vi "FPGAmain_5782_utanFIFO.vi"() -> ()   [LabVIEW 2013]
uses:
  FPGA/DataMode.ctl
  FPGA/Input_5782/5782_states.ctl
  <vilib>/Platform/TimedLoop/XDataNode/timing_clust.ctl
  <vilib>/Platform/TimedLoop/XDataNode/nitl_modes.ctl
  <vilib>/Platform/TimedLoop/XDataNode/wakeup.ctl
  <vilib>/rvi/Emulation/niFpgaSctlEmulationGetInTimedLoop.vi
  <vilib>/rvi/Emulation/niFpgaEmulationReportErrorSimple.vi
  <vilib>/rvi/Emulation/niFpgaGetClockAttributes.vi
  <vilib>/rvi/eio/common/nirviEmuTemplateMethod_errors.vi
  <vilib>/rvi/Emulation/niFpgaCriticalErrorInLSC.vi
  <vilib>/rvi/DataTransferAndStorage/Register/Emulation/niFpgaRegisterEmulationFpgaImpl.vi
  <instcachedir>/0/niFpgaRegisterEmulationFpgaImpl_DCF4BC0110594B98B44A971D60CEEC4D.lvgen/niFpgaRegisterEmulationFpgaImpl_DCF4BC0110594B98B44A971D60CEEC4D_017.vi
  <vilib>/rvi/DataTransferAndStorage/Container/Common/niFpgaContainerGetUniqueNameForEmu.vi
  <instcachedir>/0/niFpgaRegisterEmulationFpgaImpl_DCF4BC0110594B98B44A971D60CEEC4D.lvgen/niFpgaRegisterEmulationFpgaImpl_DCF4BC0110594B98B44A971D60CEEC4D_003.vi
  <instcachedir>/0/niFpgaRegisterEmulationFpgaImpl_DCF4BC0110594B98B44A971D60CEEC4D.lvgen/niFpgaRegisterEmulationFpgaImpl_DCF4BC0110594B98B44A971D60CEEC4D_016.vi
  <instcachedir>/0/niFpgaRegisterEmulationFpgaImpl_DCF4BC0110594B98B44A971D60CEEC4D.lvgen/niFpgaRegisterEmulationFpgaImpl_DCF4BC0110594B98B44A971D60CEEC4D_010.vi
  <instcachedir>/0/niFpgaRegisterEmulationFpgaImpl_DCF4BC0110594B98B44A971D60CEEC4D.lvgen/niFpgaRegisterEmulationFpgaImpl_DCF4BC0110594B98B44A971D60CEEC4D_011.vi
  <instcachedir>/0/niFpgaRegisterEmulationFpgaImpl_DCF4BC0110594B98B44A971D60CEEC4D.lvgen/niFpgaRegisterEmulationFpgaImpl_DCF4BC0110594B98B44A971D60CEEC4D_012.vi
  <instcachedir>/0/niFpgaRegisterEmulationFpgaImpl_DCF4BC0110594B98B44A971D60CEEC4D.lvgen/niFpgaRegisterEmulationFpgaImpl_DCF4BC0110594B98B44A971D60CEEC4D_009.vi
  <vilib>/rvi/interface/RandomDataEmulation/nirviRandomDataMultiElementFPGAFIFO.vi
  <instcachedir>/0/nirviRandomDataMultiElementFPGAFIFO_F2B80EDE0D7944A08478D8D26097D4DB.lvgen/nirviRandomDataMultiElementFPGAFIFO_F2B80EDE0D7944A08478D8D26097D4DB_005.vi
  <vilib>/rvi/interface/RandomDataEmulation/niFpgaRandomDataHandleErrors.vi
  <instcachedir>/0/niFpgaRegisterEmulationFpgaImpl_DCF4BC0110594B98B44A971D60CEEC4D.lvgen/niFpgaRegisterEmulationFpgaImpl_DCF4BC0110594B98B44A971D60CEEC4D_013.vi
  <vilib>/rvi/interface/RandomDataEmulation/nirviRandomDataFPGAFIFO.vi
  <instcachedir>/0/niFpgaRegisterEmulationFpgaImpl_DCF4BC0110594B98B44A971D60CEEC4D.lvgen/niFpgaRegisterEmulationFpgaImpl_DCF4BC0110594B98B44A971D60CEEC4D_018.vi
  <instcachedir>/0/niFpgaRegisterEmulationFpgaImpl_DCF4BC0110594B98B44A971D60CEEC4D.lvgen/niFpgaRegisterEmulationFpgaImpl_DCF4BC0110594B98B44A971D60CEEC4D_019.vi
  <vilib>/Platform/TimedLoop/XDataNode/XDataNode.xnode
  <vilib>/eio/EIONode/EIONode.xnode
  <vilib>/rvi/DataTransferAndStorage/Container/XNode/niFpgaContainer.xnode
  <vilib>/rvi/DataTransferAndStorage/Register/Emulation/niFpgaRegisterEmulation.vi
  <vilib>/rvi/interface/RandomDataEmulation/nirviRandomDataFpgaMultiElementTemplate.vi
  <vilib>/rvi/interface/RandomDataEmulation/nirviRandomDataFpgaReadWriteTemplate.vi
  <vilib>/Platform/TimedLoop/XDataNode/XDNodeRunTimeDep.lvlib
  <vilib>/rvi/FIFO/Fifo_Resource/nirvififoEmulationRead.vi
  <vilib>/rvi/FIFO/Fifo_Resource/nirvififoEmulationWrite.vi
panel:
  in  "Data array":fxp<+/-,16,14>[](array[numeric])=[0.0, 0.0, 0.0, 0.0]
  in  "AM phase":fxp<+,64,64>
  in  "delay phase":fxp<+,64,64>
  in  "User Command Commit":bool
  in  "User Command":u8
  out "User Command Idle":bool
  out "User Command Status":u8
  in  "User Data 0":u8
  in  "User Data 1":u8
  out "PLL Locked":bool
  out "User Error":bool
  out "Configured?":bool
  in  "Continuous":bool
  in  "5782 record length":u16=4000 caption="Samples Per Trigger" min=1 step=1
  in  "Trigger Acquisition":bool
  out "IO Module\\Trigger Input":bool
  in  "Downsample":fxp<+,8,8>=1.0
  in  "new coeffs":bool
  in  "FIR coeffs":fxp<+/-,18,18>[](array[numeric])
  in  "CIC Gain":fxp<+/-,32,1>=0.00390625 format="%#_32g"
  in  "Acquisition running":bool
  in  "Phase output":fxp<+,64,64>[](array[numeric])=[0.0, 0.0, 0.0, 0.0, 0.0, 0.0, 0.0, 0.0]
  in  "Simulated phase 5782":fxp<+,64,64>[](array[numeric])=[0.0, 0.0]
  in  "Mode":T1
  in  "Phase 5782":fxp<+,64,64>[](array[numeric])=[0.0, 0.0]
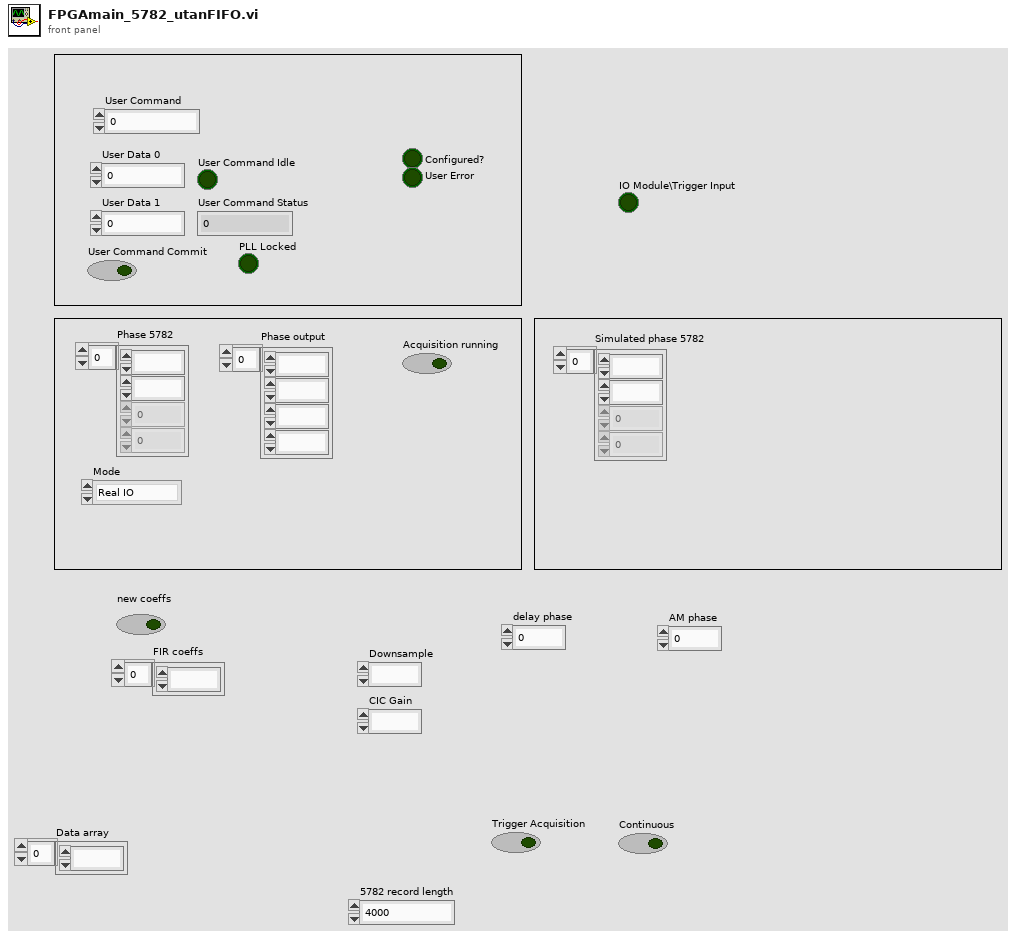
[diagram p1: front panel]
types:
  T1 = typedef "DataMode.ctl" = enum16{"Real IO", "Simulated"}
  T2 = typedef "5782_states.ctl" = enum8{"Wait for trigger", "Acquisition", "Send record length", "Quiet period"}
  T3 = typedef "XDNodeRunTimeDep.lvlib/timing_clust.ctl" = cluster{"Expected End [f-1]":u64, "Actual End [f-1]":u64, "Finished Late? [f-1]":bool, "Expected End [i-1]":u64, "Actual End [i-1]":u64, "Finished Late? [i-1]":bool, "Expected Start [i]":u64, "Actual Start [i]":u64, "Expected Start [f]":u64, "Actual Start [f]":u64, "Source Name":string, "Structure Name":string, "Period":i64, "Deadline":i64, "Offset":i64, "Start":i64, "Priority":i32, "Timeout":i32, "Mode":T4, "Wakeup Reason":T5, "Error":errorcluster, "Source Type":string, "Secondary Source Type":string, "Global End Time":u64, "Global Start Time":u64, "Frame Duration":u64, "Iteration Duration":u64, "Assigned CPU":i32, "I/O Scan Engine Mode":u32}
  T4 = typedef "XDNodeRunTimeDep.lvlib/nitl_modes.ctl" = enum32{"No Change", "Process missed periods, maintain original phase", "Discard missed periods, maintain original phase", "Process missed periods, ignore original phase", "Discard missed periods, ignore original phase"}
  T5 = typedef "XDNodeRunTimeDep.lvlib/wakeup.ctl" = enum32{"Normal", "Aborted", "Asynchronous wakeup", "Timing source error", "Timed loop error", "Timeout"}
  T6 = typedef "I16 array size 2.ctl" = i16[]
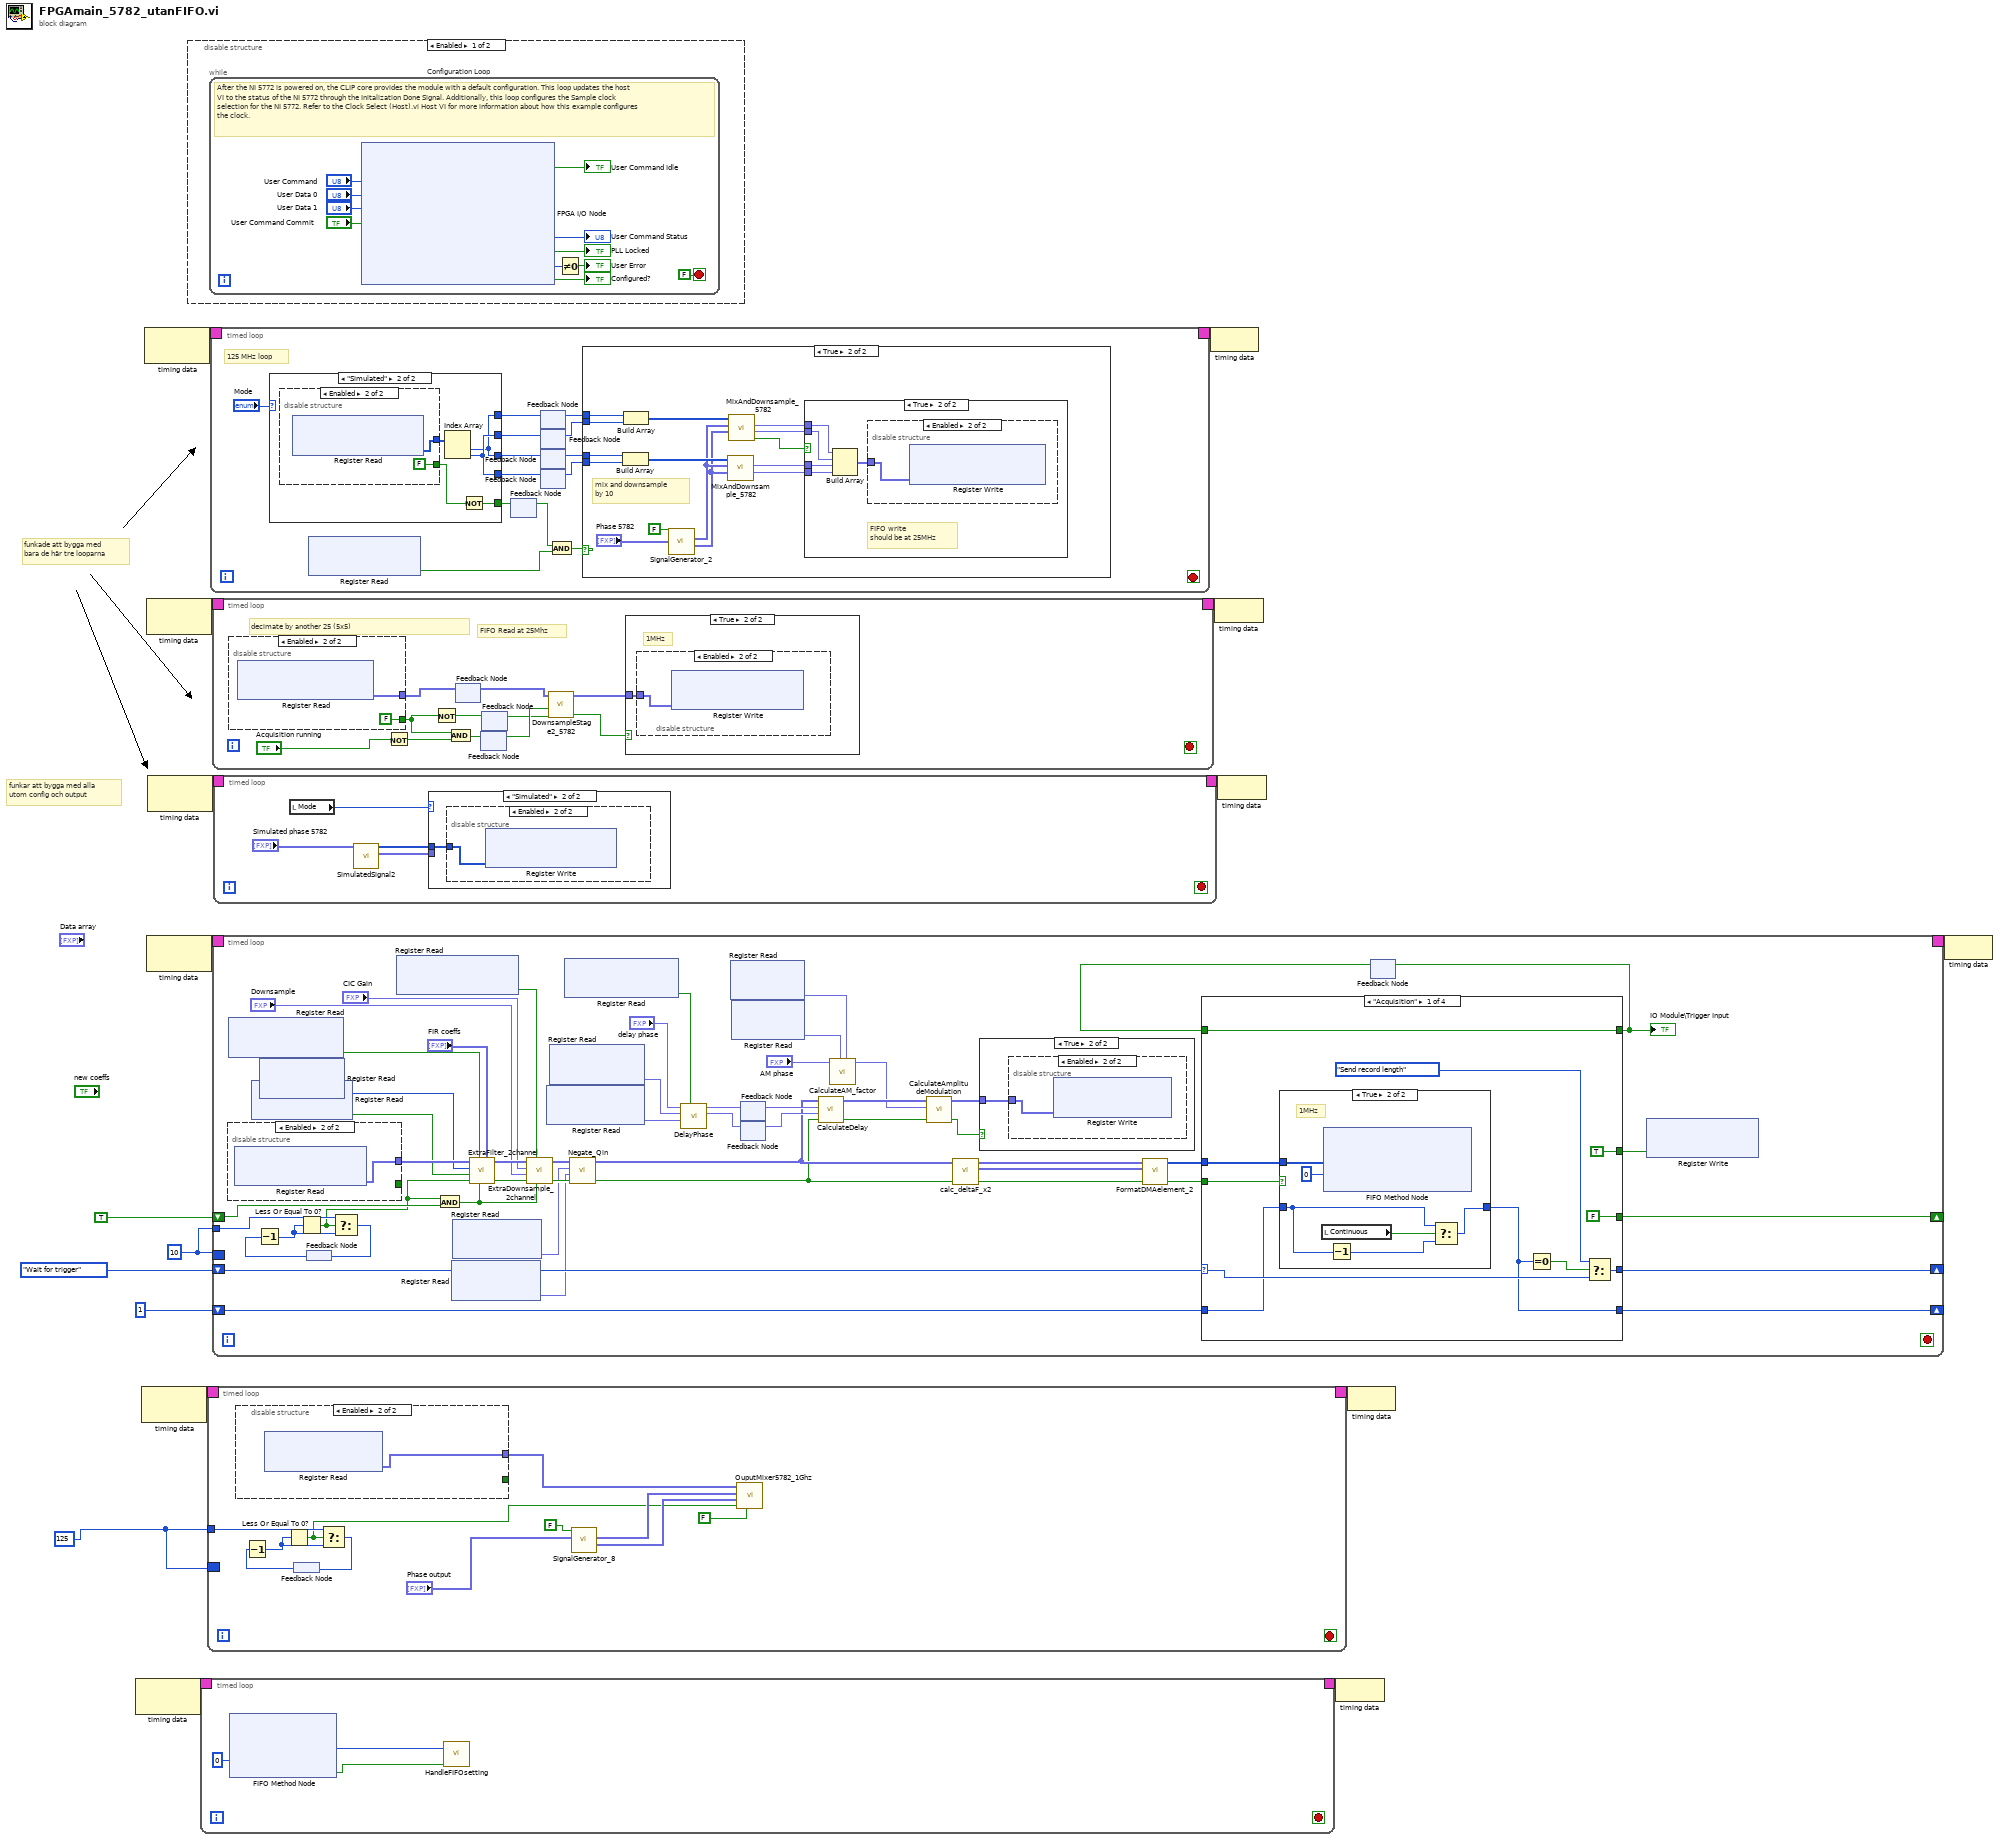
[diagram p0: block diagram]
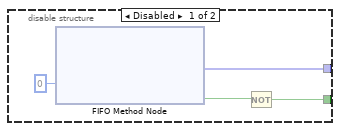
[diagram p2: hidden frame]
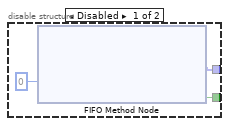
[diagram p3: hidden frame]
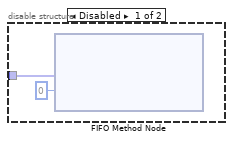
[diagram p5: hidden frame]
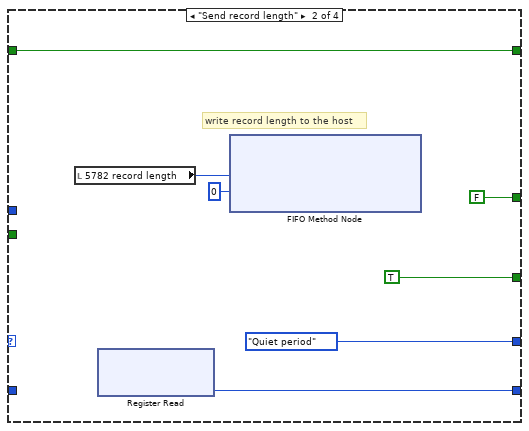
[diagram p7: hidden frame]
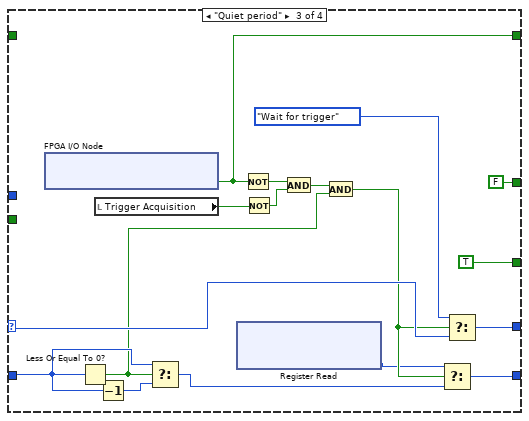
[diagram p8: hidden frame]
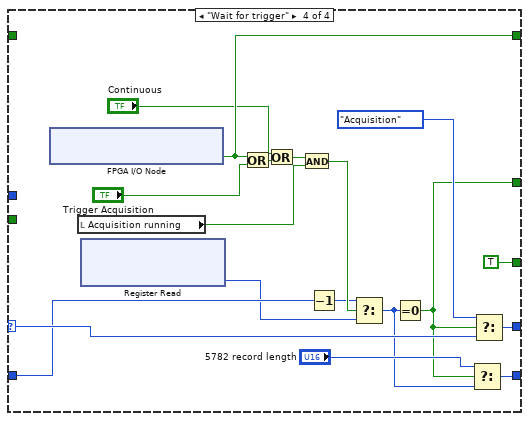
[diagram p9: hidden frame]
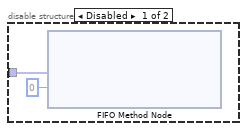
[diagram p13: hidden frame]
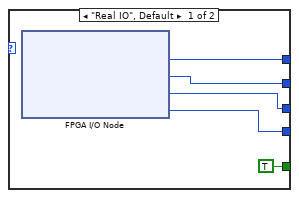
[diagram p14: hidden frame]
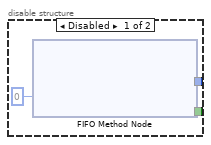
[diagram p15: hidden frame]
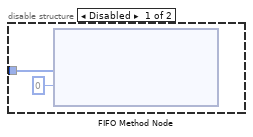
[diagram p17: hidden frame]
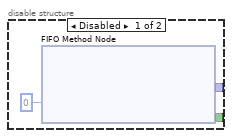
[diagram p18: hidden frame]
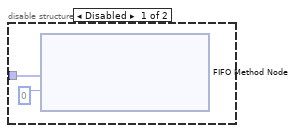
[diagram p20: hidden frame]
diagram:
  w1 = u8 125 ("trigger samples")
  w2 = u8 10 ("trigger samples")
  # "funkar att bygga med alla\nutom config och output"
  # "funkade att bygga med\nbara de här tre looparna"
  n1 = node-c288() -> (w6:T3)  [unwired: 1 in]
  n2 = node-c288() -> (w4:T3)  [unwired: 1 in]
  n3 = node-c288() -> (w13:T3)  [unwired: 1 in]
  n4 = node-c288() -> (w17:T3)  [unwired: 1 in]
  n5 = node-c288() -> (w11:T3)  [unwired: 1 in]
  n6 = node-c288() -> (w15:T3)  [unwired: 1 in]
  n7 = disable-structure shown="Enabled" {
    frame Enabled {
      n8 = while "Configuration Loop" {
        stop <- FALSE stop-if-true
        # "After the NI 5772 is powered on, the CLIP core provides the module with a default configuration. This loop updates the host VI to the status of the NI 5772 through the Initalization Done Signal. Additionally, this loop configures the Sample clock selection for the NI 5772. Refer to the Clock Select (Host).vi Host VI for more information about how this example configures the clock."
        n9 = xnode "FPGA I/O Node"("IO Module\\User Command"="User Command", "IO Module\\User Data 0"="User Data 0", "IO Module\\User Data 1"="User Data 1", "IO Module\\User Command Commit"="User Command Commit") -> ("IO Module\\User Command Idle"=→"User Command Idle":bool, "IO Module\\User Command Status"=→"User Command Status":u8, "IO Module\\PLL Locked"=→"PLL Locked":bool, "IO Module\\User Error"=w23:u8, "IO Module\\Initialization Done"=→"Configured?":bool)  [unwired: 9 in, 9 out]
        n10 = Not Equal To 0?(x=w23) -> (x != 0?=→"User Error":bool)
      }
    }
    frame Disabled {
    }
  }
  n11 = timed-loop {
    timing: w6 -> [_]
    timing-out: [_] -> w5
    stop <- _ stop-if-true
    n12 = xnode ("FIFO Method Node")("Timeout"=0) -> ("Element"=w30:u64, "Timed Out?"=w29:bool)  [unwired: 1 in, 1 out]
    n13 = call "HandleFIFOsetting.vi"("timed out"=w29, "Value"=w30) -> ()  [unwired: 10 in]
  }
  n14 = timed-loop {
    timing: w4 -> [_]
    timing-out: [_] -> w3
    tunnel: w1 -> [w38]
    border: w1 -> [_]
    stop <- _ stop-if-true
    n15 = disable-structure shown="Enabled" {
      disable-tunnel: [w47 w49] -> w42
      disable-tunnel: [w45 _] -> _
      frame Disabled {
        n16 = xnode ("FIFO Method Node")("Timeout"=0) -> ("Element"=w47:fxp<+/-,16,14>[], "Timed Out?"=w46:bool)  [unwired: 1 in, 1 out]
        n17 = Not(x=w46) -> (.not. x?=w45:bool)
      }
      frame Enabled {
        n18 = xnode ("Register Read")() -> ("Data"=w49:fxp<+/-,16,14>[])  [unwired: 1 in, 1 out]
      }
    }
    n19 = feedback #1() -> (w36:u8)
    n20 = Decrement(x=w36) -> (x-1=w34:u8)
    n21 = Less Or Equal To 0?(x=w34) -> (x <= 0?=w35:bool)
    n22 = Select(t=w38, s=w35, f=w34) -> (s? t:f=w37:u8)
    n23 = feedback-in #1(w37) -> ()
    n24 = call "SignalGenerator_8.vi"("Phase"="Phase output", "reset"=FALSE) -> ("Sine out"=w39:fxp<+/-,16,0>[], "Cosine out"=w40:fxp<+/-,16,0>[])  [unwired: 8 in]
    n25 = call "OuputMixer5782_1Ghz.vi"("reset"=FALSE, "valid in"=w35, "Sine in"=w39, "Cosine in"=w40, "Data in"=w42) -> ()  [unwired: 5 in, 2 out]
  }
  n26 = timed-loop {
    timing: w13 -> [_]
    timing-out: [_] -> w12
    stop <- _ stop-if-true
    # "125 MHz loop"
    n27 = case shown="\"Simulated\"" "Mode" {
      tunnel: [w92 w95] -> w62
      tunnel: [w91 w96] -> w60
      tunnel: [w90 w95] -> w58
      tunnel: [w89 w96] -> w55
      tunnel: [TRUE w93] -> w54
      frame "Real IO", Default {
        n28 = xnode "FPGA I/O Node"() -> ("IO Module\\AI 0 N-1"=w92:i16, "IO Module\\AI 0 N"=w91:i16, "IO Module\\AI 1 N-1"=w90:i16, "IO Module\\AI 1 N"=w89:i16)  [unwired: 4 in, 4 out]
      }
      frame "Simulated" {
        n29 = disable-structure shown="Enabled" {
          disable-tunnel: [w99 w102] -> w97
          disable-tunnel: [w98 FALSE ("Timed Out?")] -> w94
          frame Disabled {
            n30 = xnode ("FIFO Method Node")("Timeout"=0) -> ("Element"=w99:i16[], "Timed Out?"=w98:bool)  [unwired: 1 in, 1 out]
          }
          frame Enabled {
            n31 = xnode "Register Read"() -> ("Data"=w102:i16[])  [unwired: 1 in, 1 out]
          }
        }
        n32 = Index Array(array=w97) -> (element #1=w95:i16, element #2=w96:i16)  [unwired: 2 in]
        n33 = Not(x=w94) -> (.not. x?=w93:bool)
      }
    }
    n34 = xnode ("Register Read")() -> ("Data"=w52:bool)  [unwired: 1 in, 1 out]
    n35 = feedback #2() -> (w53:bool)  [unwired: 1 in]
    n36 = feedback-in #2(w54) -> ()
    n37 = feedback #3() -> (w61:i16)  [unwired: 1 in]
    n38 = feedback-in #3(w62) -> ()
    n39 = feedback #4() -> (w59:i16)  [unwired: 1 in]
    n40 = feedback-in #4(w60) -> ()
    n41 = feedback #5() -> (w57:i16)  [unwired: 1 in]
    n42 = feedback-in #5(w58) -> ()
    n43 = feedback #6() -> (w56:i16)  [unwired: 1 in]
    n44 = feedback-in #6(w55) -> ()
    n45 = And(x=w53, y=w52) -> (x .and. y?=w63:bool)
    n46 = case shown="True" w63 {
      tunnel: w61 -> [_ w70]
      tunnel: w59 -> [_ w69]
      tunnel: w57 -> [_ w68]
      tunnel: w56 -> [_ w67]
      frame False {
      }
      frame True {
        # "mix and downsample\nby 10"
        n47 = Build Array(w68, w67) -> (w79:i16[])
        n48 = Build Array(w70, w69) -> (w66:i16[])
        n49 = call "SignalGenerator_2.vi"("Phase"="Phase 5782", "reset"=FALSE) -> ("Sine out"=w71:fxp<+/-,16,0>[], "Cosine out"=w72:fxp<+/-,16,0>[])  [unwired: 8 in]
        n50 = call "MixAndDownsample_5782.vi"("Sine in"=w71, "Cosine in"=w72, "Signal Input"=w79) -> ("Q out"=w74:fxp<+/-,16,14>, "I out"=w75:fxp<+/-,16,14>)  [unwired: 6 in, 1 out]
        n51 = call "MixAndDownsample_5782.vi"("Sine in"=w71, "Cosine in"=w72, "Signal Input"=w66) -> ("data valid"=w76:bool, "Q out"=w77:fxp<+/-,16,14>, "I out"=w78:fxp<+/-,16,14>)  [unwired: 6 in]
        n52 = case shown="True" w76 {
          tunnel: w77 -> [_ w84]
          tunnel: w78 -> [_ w82]
          tunnel: w75 -> [_ w81]
          tunnel: w74 -> [_ w80]
          frame False {
          }
          frame True {
            # "FIFO write\nshould be at 25MHz"
            n53 = Build Array(w82, w84, w81, w80) -> (w83:fxp<+/-,16,14>[])
            n54 = disable-structure shown="Enabled" {
              disable-tunnel: w83 -> [w86 w87]
              frame Disabled {
                n55 = xnode ("FIFO Method Node")("Element"=w86, "Timeout"=0) -> ()  [unwired: 1 in, 2 out]
              }
              frame Enabled {
                n56 = xnode ("Register Write")("Data"=w87) -> ()  [unwired: 1 in, 1 out]
              }
            }
          }
        }
      }
    }
  }
  n57 = timed-loop {
    timing: w17 -> [_]
    timing-out: [_] -> w16
    stop <- _ stop-if-true
    # "FIFO Read at 25Mhz"
    # "decimate by another 25 (5x5)"
    n58 = disable-structure shown="Enabled" {
      disable-tunnel: [w117 FALSE ("Timed Out?")] -> w112
      disable-tunnel: [w116 w120] -> w110
      frame Disabled {
        n59 = xnode ("FIFO Method Node")("Timeout"=0) -> ("Element"=w116:fxp<+/-,16,14>[], "Timed Out?"=w117:bool)  [unwired: 1 in, 1 out]
      }
      frame Enabled {
        n60 = xnode ("Register Read")() -> ("Data"=w120:fxp<+/-,16,14>[])  [unwired: 1 in, 1 out]
      }
    }
    n61 = Not(x="Acquisition running") -> (.not. x?=w113:bool)
    n62 = Not(x=w112) -> (.not. x?=w106:bool)
    n63 = And(x=w112, y=w113) -> (x .and. y?=w108:bool)
    n64 = feedback #7() -> (w109:fxp<+/-,16,14>[])  [unwired: 1 in]
    n65 = feedback-in #7(w110) -> ()
    n66 = feedback #8() -> (w107:bool)  [unwired: 1 in]
    n67 = feedback-in #8(w108) -> ()
    n68 = feedback #9() -> (w105:bool)  [unwired: 1 in]
    n69 = feedback-in #9(w106) -> ()
    n70 = call "DownsampleStage2_5782.vi"("valid in"=w105, "reset"=w107, "Data in"=w109) -> ("valid out"=w114:bool, "data out"=w115:fxp<+/-,16,14>[])  [unwired: 7 in]
    n71 = case shown="True" w114 {
      tunnel: w115 -> [_ w121]
      frame False {
      }
      frame True {
        # "1MHz"
        n72 = disable-structure shown="Enabled" {
          disable-tunnel: w121 -> [w122 w124]
          frame Disabled {
            n73 = xnode ("FIFO Method Node")("Element"=w122, "Timeout"=0) -> ()  [unwired: 1 in, 2 out]
          }
          frame Enabled {
            n74 = xnode ("Register Write")("Data"=w124) -> ()  [unwired: 1 in, 1 out]
          }
        }
      }
    }
  }
  n75 = timed-loop {
    timing: w11 -> [_]
    timing-out: [_] -> w10
    shift-right: [w176] -> _
    shift-left: 5782_states."Wait for trigger" ("5782 states") -> [w178]
    shift-right: [w175] -> _
    shift-left: u16 1 ("trigger samples") -> [w177]
    shift-right: [w164] -> _
    shift-left: TRUE -> [w167]
    border: w2 -> [_]
    tunnel: w2 -> [w130]
    stop <- _ stop-if-true
    n76 = disable-structure shown="Enabled" {
      disable-tunnel: [w180 w182] -> w168
      disable-tunnel: [w179 _] -> _
      frame Disabled {
        n77 = xnode ("FIFO Method Node")("Timeout"=0) -> ("Element"=w180:fxp<+/-,16,14>[], "Timed Out?"=w179:bool)  [unwired: 1 in, 1 out]
      }
      frame Enabled {
        n78 = xnode ("Register Read")() -> ("Data"=w182:fxp<+/-,16,14>[])  [unwired: 1 in, 1 out]
      }
    }
    n79 = xnode ("Register Read")() -> ("Data"=w142:bool)  [unwired: 1 in, 1 out]
    n80 = xnode ("Register Read")() -> ("Data"=w132:bool)  [unwired: 1 in, 1 out]
    n81 = xnode ("Register Read")() -> ("Data"=w133:i32)  [unwired: 1 in, 1 out]
    n82 = feedback #10() -> (w131:u8)
    n83 = Decrement(x=w131) -> (x-1=w129:u8)
    n84 = Less Or Equal To 0?(x=w129) -> (x <= 0?=w127:bool)
    n85 = Select(t=w130, s=w127, f=w129) -> (s? t:f=w128:u8)
    n86 = feedback-in #10(w128) -> ()
    n87 = xnode ("Register Read")() -> ("Data"=w134:bool)  [unwired: 1 in, 1 out]
    n88 = And(x=w127, y=w167) -> (x .and. y?=w174:bool)
    n89 = xnode ("Register Read")() -> ("Data"=w140:fxp<+/-,16,14>)  [unwired: 1 in, 1 out]
    n90 = xnode ("Register Read")() -> ("Data"=w141:fxp<+/-,16,14>)  [unwired: 1 in, 1 out]
    n91 = call "ExtraFilter_2channel.vi"(5:"new coeffs"="FIR coeffs", "reset"=w174, 7:"new coeffs"=w142, "valid in"=w127, "enable filter"=w132, "new shift"=w133, "Data in"=w168) -> ("valid out"=w173:bool, "Data out"=w172:fxp<+/-,16,14>[])  [unwired: 3 in]
    n92 = call "ExtraDownsample_2channel.vi"("reset"=w174, "Set downsample"=w134, "valid in"=w173, "Downsample"="Downsample", "CIC Gain"="CIC Gain", "Data in"=w172) -> ("valid out"=w159:bool, "Data out"=w160:fxp<+/-,16,14>[])  [unwired: 4 in]
    n93 = xnode ("Register Read")() -> ("Data"=w135:fxp<+/-,16,0>)  [unwired: 1 in, 1 out]
    n94 = xnode ("Register Read")() -> ("Data"=w136:fxp<+/-,16,0>)  [unwired: 1 in, 1 out]
    n95 = xnode ("Register Read")() -> ("Data"=w137:bool)  [unwired: 1 in, 1 out]
    n96 = call "Negate_Qin.vi"("valid in"=w159, "DC offset chan 1"=w140, "DC offset chan 0"=w141, "Data in"=w160) -> ("valid out"=w145:bool, "Data out"=w151:fxp<+/-,16,14>[])  [unwired: 6 in]
    n97 = call "DelayPhase.vi"("Use fixed delay"=w137, "fixed cos_fi"=w135, "fixed sin fi"=w136, "delay phase"="delay phase") -> ("cos_fi"=w148:fxp<+/-,16,0>, "sin fi"=w149:fxp<+/-,16,0>)  [unwired: 6 in]
    n98 = xnode ("Register Read")() -> ("Data"=w139:fxp<+/-,16,2>)  [unwired: 1 in, 1 out]
    n99 = xnode ("Register Read")() -> ("Data"=w138:fxp<+/-,16,2>)  [unwired: 1 in, 1 out]
    n100 = feedback-in #11(w149) -> ()
    n101 = feedback #11() -> (w158:fxp<+/-,16,0>)  [unwired: 1 in]
    n102 = feedback #12() -> (w157:fxp<+/-,16,0>)  [unwired: 1 in]
    n103 = feedback-in #12(w148) -> ()
    n104 = call "CalculateDelay.vi"("input valid"=w145, "cos_fi"=w157, "sin fi"=w158, "Data in"=w151) -> ("output valid"=w155:bool, "Data out"=w156:fxp<+/-,16,14>[])  [unwired: 6 in]
    n105 = call "CalculateAM_factor.vi"("b_am"=w139, "a_am"=w138, "AM phase"="AM phase") -> ("AM_factor"=w152:fxp<+/-,16,2>)  [unwired: 7 in, 1 out]
    n106 = call "CalculateAmplitudeModulation.vi"("input valid"=w155, "AM_factor"=w152, "Data in"=w156) -> ("output valid"=w153:bool, "Data out"=w154:fxp<+/-,16,14>[])  [unwired: 7 in]
    n107 = call "calc_deltaF_x2.vi"("valid in"=w145, "Data in"=w151) -> ("valid out"=w144:bool, "deltaF"=w143:fxp<+/-,32,30>[], "Data out"=w146:fxp<+/-,16,14>[])  [unwired: 7 in]
    n108 = case shown="True" w153 {
      tunnel: w154 -> [_ w183]
      frame False {
      }
      frame True {
        n109 = disable-structure shown="Enabled" {
          disable-tunnel: w183 -> [w184 w186]
          frame Disabled {
            n110 = xnode ("FIFO Method Node")("Element"=w184, "Timeout"=0) -> ()  [unwired: 1 in, 2 out]
          }
          frame Enabled {
            n111 = xnode ("Register Write")("Data"=w186) -> ()  [unwired: 1 in, 1 out]
          }
        }
      }
    }
    n112 = call "FormatDMAelement_2.vi"("valid in"=w144, "deltaF"=w143, "Data in"=w146) -> ("valid out"=w165:bool, "Element"=w166:u64[])  [unwired: 7 in]
    n113 = feedback #13() -> (w162:bool)  [unwired: 1 in]
    n114 = case shown="\"Acquisition\"" w178 {
      selector: w178 -> [w197 _ w227 w246]
      tunnel: w177 -> [w193 _ w215 w233]
      tunnel: [w196 5782_states."Quiet period" ("5782 states") w226 w245] -> w176
      tunnel: [w190 w205 w228 w244] -> w175
      tunnel: w166 -> [w191 _ _ _]
      tunnel: w165 -> [w192 _ _ _]
      tunnel: [FALSE TRUE TRUE TRUE] -> w164
      tunnel: [TRUE FALSE ("5782 triggered") FALSE ("5782 triggered") w237] -> w163
      tunnel: [w189 w206 w217 w236] -> w161
      tunnel: w162 -> [w189 w206 _ _]
      frame "Acquisition" {
        n115 = case shown="True" w192 {
          tunnel: w191 -> [_ w204]
          tunnel: [w198 w201] -> w190
          tunnel: w193 -> [w198 w199]
          frame False {
          }
          frame True {
            # "1MHz"
            n116 = local read "Continuous"() -> (w202:bool)
            n117 = xnode ("FIFO Method Node")("Element"=w204, "Timeout"=0) -> ()  [unwired: 1 in, 2 out]
            n118 = Decrement(x=w199) -> (x-1=w200:u16)
            n119 = Select(t=w199, s=w202, f=w200) -> (s? t:f=w201:u16)
          }
        }
        n120 = Equal To 0?(x=w190) -> (x = 0?=w194:bool)
        n121 = Select(t=5782_states."Send record length" ("5782 states"), s=w194, f=w197) -> (s? t:f=w196:T2)
      }
      frame "Send record length" {
        # "write record length to the host"
        n122 = local read "5782 record length"() -> (w208:u16)
        n123 = xnode ("Register Read")() -> ("Data"=w205:u16)  [unwired: 1 in, 1 out]
        n124 = xnode ("FIFO Method Node")("Element"=w208, "Timeout"=0) -> ()  [unwired: 1 in, 2 out]
      }
      frame "Quiet period" {
        n125 = xnode "FPGA I/O Node"() -> ("IO Module\\Trigger Input"=w217:bool)  [unwired: 1 in, 1 out]
        n126 = Less Or Equal To 0?(x=w215) -> (x <= 0?=w214:bool)
        n127 = local read "Trigger Acquisition"() -> (w223:bool)
        n128 = Decrement(x=w215) -> (x-1=w216:u16)
        n129 = Select(t=w215, s=w214, f=w216) -> (s? t:f=w213:u16)
        n130 = xnode ("Register Read")() -> ("Data"=w212:u16)  [unwired: 1 in, 1 out]
        n131 = Not(x=w217) -> (.not. x?=w222:bool)
        n132 = Not(x=w223) -> (.not. x?=w221:bool)
        n133 = And(x=w222, y=w221) -> (x .and. y?=w220:bool)
        n134 = And(x=w220, y=w214) -> (x .and. y?=w225:bool)
        n135 = Select(t=w212, s=w225, f=w213) -> (s? t:f=w228:u16)
        n136 = Select(t=5782_states."Wait for trigger" ("5782 states"), s=w225, f=w227) -> (s? t:f=w226:T2)
      }
      frame "Wait for trigger" {
        n137 = xnode "FPGA I/O Node"() -> ("IO Module\\Trigger Input"=w236:bool)  [unwired: 1 in, 1 out]
        n138 = local read "Acquisition running"() -> (w238:bool)
        n139 = xnode ("Register Read")() -> ("Data"=w229:u16)  [unwired: 1 in, 1 out]
        n140 = Or(x=w236, y="Trigger Acquisition") -> (x .or. y?=w232:bool)
        n141 = Or(x="Continuous", y=w232) -> (x .or. y?=w230:bool)
        n142 = And(x=w230, y=w238) -> (x .and. y?=w239:bool)
        n143 = Decrement(x=w233) -> (x-1=w234:u16)
        n144 = Select(t=w234, s=w239, f=w229) -> (s? t:f=w235:u16)
        n145 = Equal To 0?(x=w235) -> (x = 0?=w237:bool)
        n146 = Select(t="5782 record length", s=w237, f=w235) -> (s? t:f=w244:u16)
        n147 = Select(t=5782_states."Acquisition" ("5782 states"), s=w237, f=w246) -> (s? t:f=w245:T2)
      }
    }
    "IO Module\\Trigger Input" <- w161
    n148 = feedback-in #13(w161) -> ()
    n149 = xnode ("Register Write")("Data"=w163) -> ()  [unwired: 1 in, 1 out]
  }
  n150 = timed-loop {
    timing: w15 -> [_]
    timing-out: [_] -> w14
    stop <- _ stop-if-true
    n151 = local read "Mode"() -> (w252:T1)
    n152 = call "SimulatedSignal2.vi"("Phase"="Simulated phase 5782") -> ("dummy do not use"=w249:fxp<+/-,16,0>[], "output"=w251:T6)  [unwired: 9 in]
    n153 = case shown="\"Simulated\"" w252 {
      tunnel: w251 -> [_ w253]
      tunnel: w249 -> [_ _]
      frame "Real IO", Default {
      }
      frame "Simulated" {
        n154 = disable-structure shown="Enabled" {
          disable-tunnel: w253 -> [w254 w256]
          frame Disabled {
            n155 = xnode ("FIFO Method Node")("Element"=w254, "Timeout"=0) -> ()  [unwired: 1 in, 2 out]
          }
          frame Enabled {
            n156 = xnode "Register Write"("Data"=w256) -> ()  [unwired: 1 in, 1 out]
          }
        }
      }
    }
  }
  n157 = node-c288(w12) -> ()
  n158 = node-c288(w16) -> ()
  n159 = node-c288(w14) -> ()
  n160 = node-c288(w5) -> ()
  n161 = node-c288(w3) -> ()
  n162 = node-c288(w10) -> ()
